vi "TestCopyARGBImage.vi"(8 "error in (no error)":errorcluster, 11 "Test Case In":refnum<class "Image.lvclass">) -> (0 "error out":errorcluster, 3 "Test Case Out":refnum<class "Image.lvclass">)   [LabVIEW 2020, in "g_ar_toolkit.test.lvlib" / "Image.lvclass"]
uses:
  Image.lvclass
  C:/Program Files (x86)/National Instruments/LabVIEW 2020/vi.lib/Astemes/LUnit/Test Case.lvclass
  g_ar_toolkit/Image Size Cluster.ctl
  <vilib>/Astemes/LUnit/Test Case.lvclass/Test Case.ctl
  g_ar_toolkit/Create_Empty_Image_ARGB.vi
  4993e8ee-a06a-463a-9684-69129f64d5ce.vi
  <vilib>/Astemes/LUnit/Append Pass Result.vi
  <vilib>/Astemes/LUnit/Append Fail Result.vi
  <vilib>/Astemes/LUnit/Describe Comparison.vi
  <vilib>/Astemes/LUnit/Compare Variants.vi
  <vilib>/Astemes/LUnit/Variant to string.vi
  <vilib>/Utility/error.llb/Error Cluster From Error Code.vi
  <vilib>/picture/picture.llb/Draw Rectangle.vi
  <vilib>/picture/pictutil.llb/Picture to Pixmap.vi
  <vilib>/Utility/Data Type/Get Type Information.vi
  <vilib>/Utility/LVClass/Get LV Class Name.vi
  Image.lvclass/Image.ctl
  g_ar_toolkit.lvlib
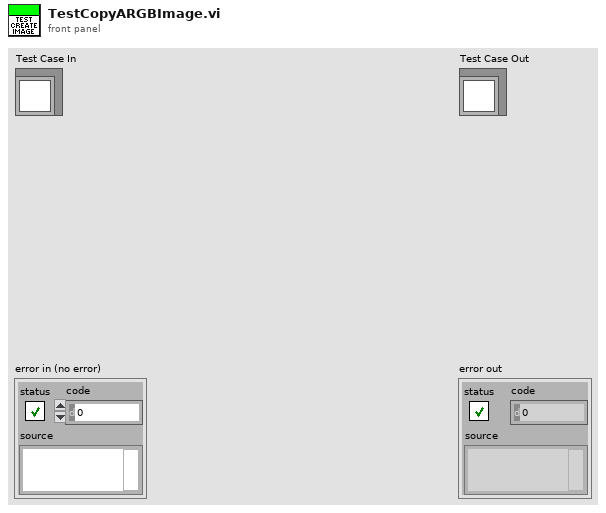
[diagram p1: front panel]
types:
  T1 = typedef "g_ar_toolkit.lvlib/Image Size Cluster.ctl" = cluster{"Width":u16, "Height":u16}
  T2 = typedef "imagedata.ctl" = cluster{"image type":i32, "image depth":i32, "image":u8[], "mask":u8[], "colors":u32[], "Rectangle":cluster{"left":i16, "top":i16, "right":i16, "bottom":i16}}
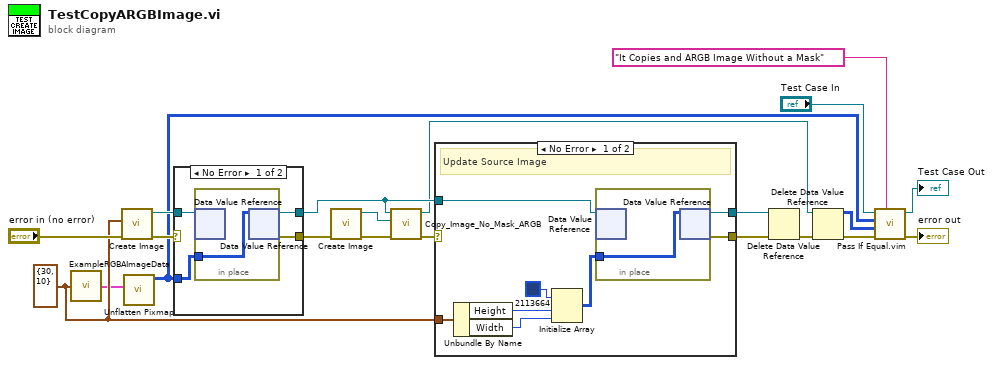
[diagram p0: block diagram]
diagram:
  w9 = T1 {"Width"=30, "Height"=10} ("Preallocated Image Size (Default - 0,0)")
  n1 = call "ExampleRGBAImageData.vi"("Image Size"=w9) -> ("RGB Image Data"=w5:T2)
  n2 = call-poly "Create Image.vi"("error in (no error)"="error in (no error)", "Preallocated Image Size (Default - 0,0)"=w9) -> ("error out"=w15:errorcluster, "New ARGB Image"=w16:refnum<data-value>)  [unwired: 8 in]
  n3 = call <vilib>:"Unflatten Pixmap.vi"("image data"=w5) -> ("24-bit pixmap"=w1:u32[][])  [unwired: 4 in, 6 out]
  n4 = case shown="No Error" w15 {
    selector: w15 -> [_ w27]
    tunnel: w16 -> [w25 w28]
    tunnel: [w24 w28] -> w7
    tunnel: [w23 w27] -> w14
    tunnel: w1 -> [w22 _]
    frame No Error {
      n5 = in-place {
        in-place-border: w22 -> [w26]
        n6 = in-place-dvr #1(w25) -> ()  [unwired: 2 out]
        n7 = in-place-dvr #1(w26) -> (w24:refnum<data-value>, w23:errorcluster)
      }
    }
    frame Error {
    }
  }
  n8 = call-poly "Create Image.vi"("error in (no error)"=w14) -> ("error out"=w12:errorcluster, "New ARGB Image"=w13:refnum<data-value>)  [unwired: 9 in]
  n9 = call "Copy_Image_No_Mask_ARGB.vi"("error in (no error)"=w12, "ARGB Image Destination"=w13, "ARGB Image Source"=w7) -> ("error out"=w8:errorcluster, "ARGB Image Destination (duplicate)"=w3:refnum<data-value>)  [unwired: 7 in]
  n10 = case shown="No Error" w8 {
    selector: w8 -> [_ w38]
    tunnel: w7 -> [w36 w39]
    tunnel: [w35 w39] -> w4
    tunnel: [w34 w38] -> w6
    tunnel: w9 -> [w31 _]
    frame No Error {
      # "Update Source Image"
      n11 = Unbundle By Name(w31) -> ("Height"=w33:u16, "Width"=w32:u16)
      n12 = Initialize Array(u32 2113664, w33, w32) -> (w29:u32[][])
      n13 = in-place {
        in-place-border: w29 -> [w37]
        n14 = in-place-dvr #2(w36) -> ()  [unwired: 2 out]
        n15 = in-place-dvr #2(w37) -> (w35:refnum<data-value>, w34:errorcluster)
      }
    }
    frame Error {
    }
  }
  n16 = Delete Data Value Reference(data value reference=w4, error in=w6) -> (error out=w11:errorcluster)  [unwired: 1 out]
  n17 = Delete Data Value Reference(data value reference=w3, error in=w11) -> (data value=w2:u32[][], error out=w10:errorcluster)
  n18 = call "Pass If Equal.vim"("Description"="It Copies and ARGB Image Without a Mask", "error in (no error)"=w10, "Actual"=w2, "Expected"=w1, "LUnit Test Case In"="Test Case In") -> ("error out"=→"error out":errorcluster, "LUnit Test Case Out"=→"Test Case Out":refnum<class "Image.lvclass">)  [unwired: 5 in]
